vi "test-ltv-differential-drive-controller-Test1.vi"() -> (3 "All tests passed":bool)   [LabVIEW 2019]
uses:
  <vilib>/Rock Robotics/WPI/ThirdParty/JAS_Junk/TrajLib/TRAJ_STATE.ctl
  <vilib>/Rock Robotics/WPI/ThirdParty/JAS_Junk/TrajLib/POSE2D.ctl
  <vilib>/Rock Robotics/WPI/ThirdParty/JAS_Junk/TrajLib/TRANSLATION2D.ctl
  <vilib>/Rock Robotics/WPI/ThirdParty/JAS_Junk/TrajLib/ROTATION2D.ctl
  <vilib>/Rock Robotics/WPI/ThirdParty/JAS_Junk/TrajLib/LINEAR_SYSTEM.ctl
  <vilib>/Analysis/Matrix/Datatypes/RealMatrix.ctl
  <vilib>/Rock Robotics/WPI/ThirdParty/JAS_Junk/TrajLib/LTV_DIFF_DRIVE_CTRL.ctl
  <vilib>/Rock Robotics/WPI/ThirdParty/JAS_Junk/TrajLib/FUNCTION_GENERATOR_MATRIX.ctl
  <vilib>/Rock Robotics/WPI/ThirdParty/JAS_Junk/TrajLib/TRAJECTORY_SPLINE_TYPE_ENUM.ctl
  <vilib>/numeric/Random Number (Range) DBL.vi
  <vilib>/Rock Robotics/WPI/ThirdParty/JAS_Junk/TrajLib/Conv_Inches_Meters.vi
  <vilib>/Rock Robotics/WPI/ThirdParty/JAS_Junk/TrajLib/Rotation2d_CreateAngle.vi
  <vilib>/Rock Robotics/WPI/ThirdParty/JAS_Junk/TrajLib/Translation2d_Create.vi
  <vilib>/Rock Robotics/WPI/ThirdParty/JAS_Junk/TrajLib/MatBuilder_Create.vi
  <vilib>/Rock Robotics/WPI/ThirdParty/JAS_Junk/TrajLib/LinearSystem_New.vi
  <vilib>/Rock Robotics/WPI/ThirdParty/JAS_Junk/TrajLib/MatrixHelper_Zero.vi
  <vilib>/Rock Robotics/WPI/ThirdParty/JAS_Junk/TrajLib/MatBuilder_Fill.vi
  <vilib>/Rock Robotics/WPI/ThirdParty/JAS_Junk/TrajLib/MatrixHelper_CoerceSize.vi
  <vilib>/Analysis/Matrix/Numeric/Add/Add - RM,RM.vi
  <vilib>/Rock Robotics/WPI/ThirdParty/JAS_Junk/TrajLib/Trajectory_Library.lvlib
  <vilib>/Analysis/Matrix/NI_Matrix.lvlib
panel:
  out "Error Graph":dbl[][](graph)
  out "DiffDriveCtrl":T1
  out "Output":T3
  out "Return X":T3
  out "Time":dbl=-1.0
  out "Create Error":bool
  out "Linearsystem":T4
  out "Error":bool
  out "Max\nIterationCount":i32
  out "Any Calc Error":bool
  out "Output Graph":dbl[][](graph)
  out "XY Graph":cluster{dbl[], dbl[]}[](graph)
  out "X":bool
  out "Y":bool
  out "Rot":bool
  out "TotalTime_Sec":dbl
  out "Calc Error":bool
  out "TrajStatePose":T5={"TRANSLATION"={"X"=0.0, "Y"=0.0}, "ROTATION"={"VALUE"=0.0, "COS"=1.0, "SIN"=0.0}} {"ROTATION"."SIN" format="%13.4f"; "ROTATION"."COS" format="%13.4f"; "ROTATION"."VALUE" format="%13.4f"; "TRANSLATION"."Y" format="%14.3f"; "TRANSLATION"."X" format="%14.3f"}
  out "UpdatedPose":T5 {"ROTATION"."SIN" format="%13.4f"; "ROTATION"."COS" format="%13.4f"; "ROTATION"."VALUE" format="%13.4f"; "TRANSLATION"."Y" format="%14.3f"; "TRANSLATION"."X" format="%14.3f"}
  out "OutputTRAJ_STATE":T8={"TimeSeconds"=0.0, "Velocity"=0.0, "Acceleration"=0.0, "POSE"={"TRANSLATION"={"X"=0.0, "Y"=0.0}, "ROTATION"={"VALUE"=0.0, "COS"=1.0, "SIN"=0.0}}, "Curvature"=0.0} {"POSE"."ROTATION"."SIN" format="%13.4f"; "POSE"."ROTATION"."COS" format="%13.4f"; "POSE"."ROTATION"."VALUE" format="%13.4f"; "POSE"."TRANSLATION"."Y" format="%14.3f"; "POSE"."TRANSLATION"."X" format="%14.3f"}
  out "At Reference":bool
  in  "Use Noise":bool
  in  "Use Output Limit":bool=TRUE
  # "< 5, 1 >"
  # "< 2 1 >"
  # "<States,States>"
  # "<States,Inputs>"
  # "<Outputs,States>"
  # "<Outputs,Inputs>"
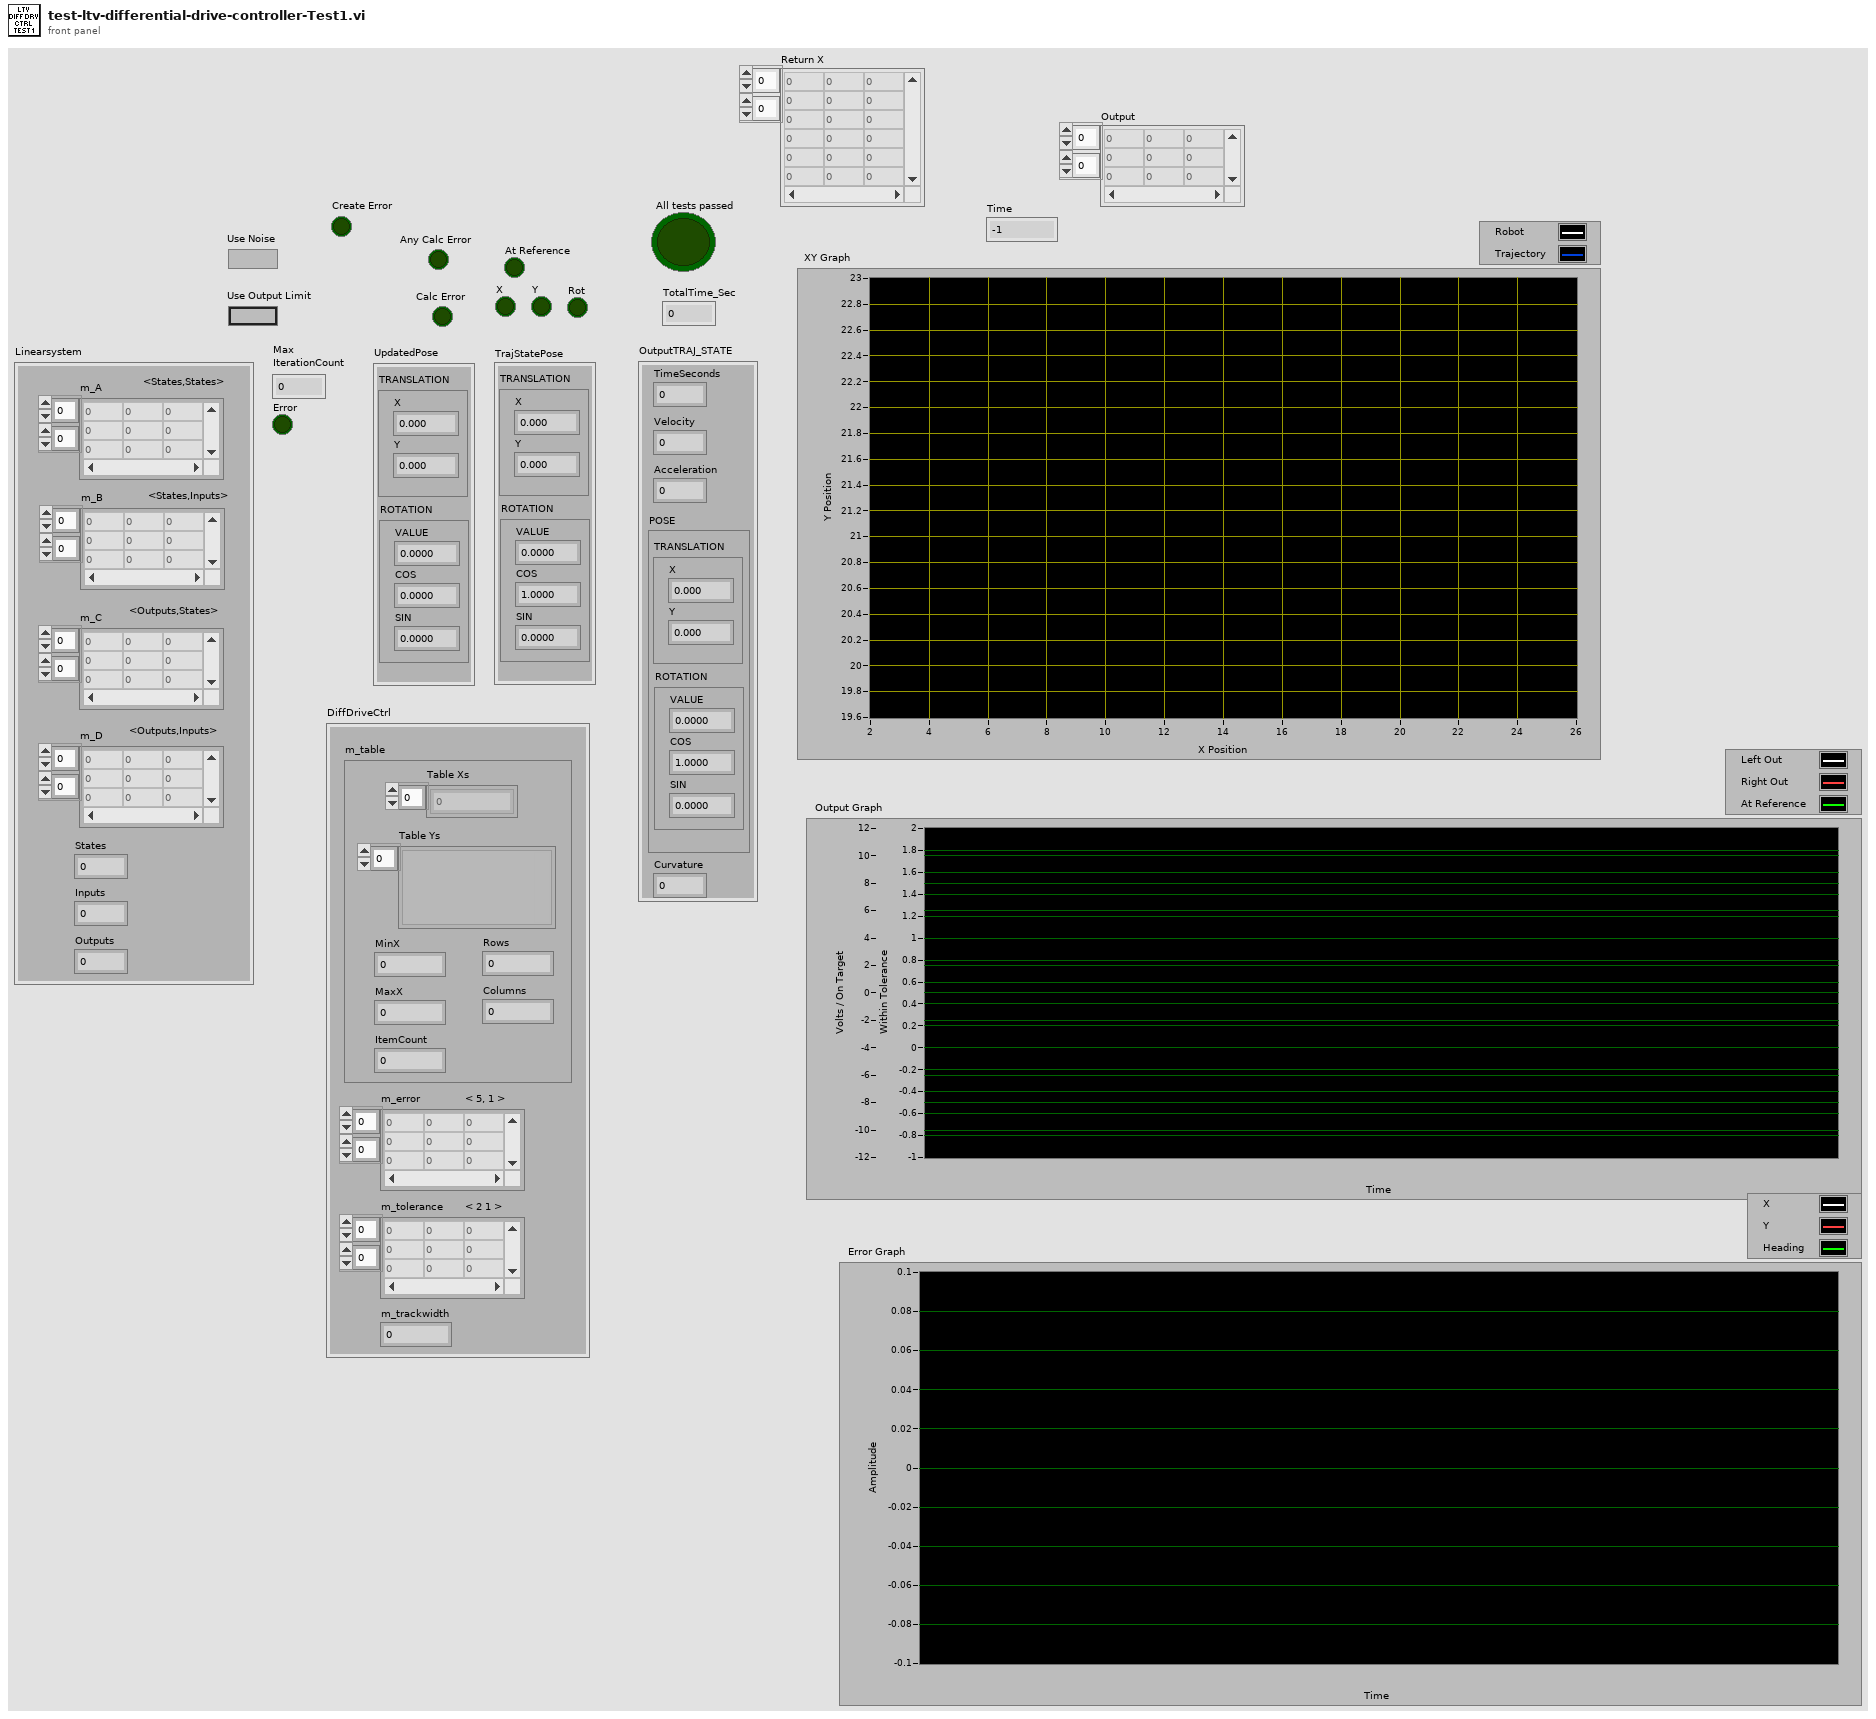
[diagram p1: front panel]
types:
  T1 = typedef "Trajectory_Library.lvlib/LTV_DIFF_DRIVE_CTRL.ctl" = cluster{"m_table":T2, "m_error":T3, "m_tolerance":T3, "m_trackwidth":dbl}
  T2 = typedef "Trajectory_Library.lvlib/FUNCTION_GENERATOR_MATRIX.ctl" = cluster{"Table Xs":dbl[], "Table Ys":variant[], "MinX":dbl, "MaxX":dbl, "ItemCount":i32, "Rows":i32, "Columns":i32}
  T3 = typedef "NI_Matrix.lvlib/RealMatrix.ctl" = dbl[][]
  T4 = typedef "Trajectory_Library.lvlib/LINEAR_SYSTEM.ctl" = cluster{"m_A":T3, "m_B":T3, "m_C":T3, "m_D":T3, "States":i32, "Inputs":i32, "Outputs":i32}
  T5 = typedef "Trajectory_Library.lvlib/POSE2D.ctl" = cluster{"TRANSLATION":T6, "ROTATION":T7}
  T6 = typedef "Trajectory_Library.lvlib/TRANSLATION2D.ctl" = cluster{"X":dbl, "Y":dbl}
  T7 = typedef "Trajectory_Library.lvlib/ROTATION2D.ctl" = cluster{"VALUE":dbl, "COS":dbl, "SIN":dbl}
  T8 = typedef "Trajectory_Library.lvlib/TRAJ_STATE.ctl" = cluster{"TimeSeconds":dbl, "Velocity":dbl, "Acceleration":dbl, "POSE":T5, "Curvature":dbl}
  T9 = typedef "Trajectory_Library.lvlib/TRAJECTORY_SPLINE_TYPE_ENUM.ctl" = enum16{"Cubic", "Cubic With Weights", "Quintic", "Quintic With Weights"}
  T10 = typedef "Trajectory_Library.lvlib/WEIGHTED_WAYPOINT.ctl" = cluster{"TRANSLATION":T6, "ROTATION":T7, "SCALAR":dbl}
  T11 = typedef "Trajectory_Library.lvlib/TRAJ_CONFIG.ctl" = cluster{"MaxVelocity":dbl, "Max Acceleration":dbl, "StartVelocity":dbl, "End Velocity":dbl, "Reversed":bool, "DiffDrKineConstntDefined":bool, "CentAcellConstntDefined":bool, "DiffDrVoltConstntDefined":bool, "DIFF_DRIVE_KINE_CONSTRAINT":T12, "CENTRIPETAL_ACCEL_CONSTRAINT":T14, "SwerveDrKineConstntDefined":bool, "SWERVE_DRIVE_KINE_CONSTRAINT":T15, "DIFF_DRIVE_VOLTAGE_CONSTRAINT":T17, "MECANUM_DRIVE_KINE_CONSTRAINT":T19, "MecanumDrKineConstntDefined":bool}
  T12 = typedef "Trajectory_Library.lvlib/TRAJ_CONSTRAINT_DIIF_DRIVE_KINEMATICS.ctl" = cluster{"Max Speed (M/S)":dbl, "DIFF_DRIVE_KINEMATICS":T13, "Max Accel (M/S2)":dbl}
  T13 = typedef "Trajectory_Library.lvlib/DIFF_DRIVE_KINEMATICS.ctl" = cluster{"TrackWidth_Meters":dbl}
  T14 = typedef "Trajectory_Library.lvlib/TRAJ_CONSTRAINT_CENTRIPETAL_ACCEL.ctl" = cluster{"Max Cent Accel":dbl}
  T15 = typedef "Trajectory_Library.lvlib/TRAJ_CONSTRAINT_SWERVE_DRIVE_KINEMATICS.ctl" = cluster{"Max Speed (M/S)":dbl, "SwerveKinematics":T16}
  T16 = typedef "Trajectory_Library.lvlib/SWERVE_DRIVE_KINEMATICS.ctl" = cluster{"NumModules":i32, "InverseKinematics":T3, "ForwardKinematics":T3, "Modules":T6[], "PrevCoR":T6}
  T17 = typedef "Trajectory_Library.lvlib/TRAJ_CONSTRAINT_DIIF_DRIVE_VOLTAGE.ctl" = cluster{"Max Voltage":dbl, "DIFF_DRIVE_KINEMATICS":T13, "SIMPLE_MOTOR_FF":T18}
  T18 = typedef "Trajectory_Library.lvlib/SIMPLE_MOTOR_FF.ctl" = cluster{"Ks":dbl, "Kv":dbl, "Ka":dbl}
  T19 = typedef "Trajectory_Library.lvlib/TRAJ_CONSTRAINT_MECA_DRIVE_KINEMATICS.ctl" = cluster{"Max Speed (M/S)":dbl, "MECA_DRIVE_KINEMATICS":T20}
  T20 = typedef "Trajectory_Library.lvlib/MECA_DRIVE_KINEMATICS.ctl" = cluster{"FrontLeft":T6, "FrontRight":T6, "RearLeft":T6, "RearRight":T6, "InverseKinematics":T3, "ForwardKinematics":T3, "PrevCoR":T6}
  T21 = typedef "Trajectory_Library.lvlib/TRAJECTORY.ctl" = cluster{"TotalTImeSecs":dbl, "States":T8[]}
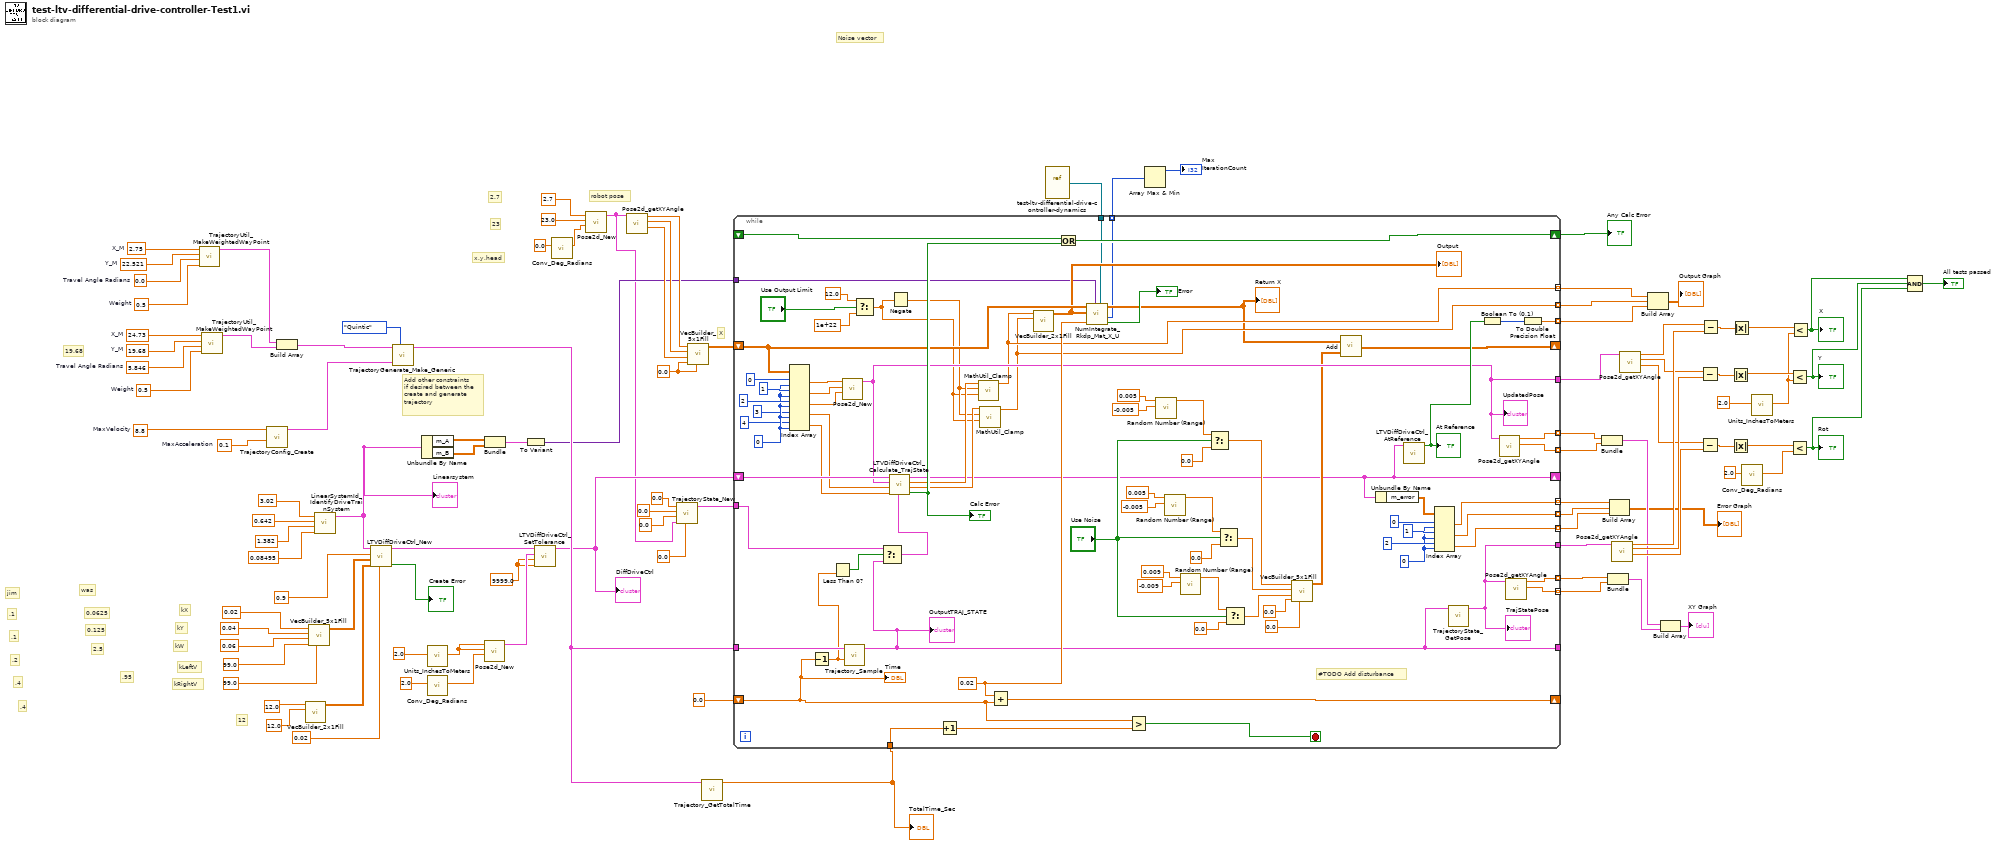
[diagram p0: block diagram]
diagram:
  w15 = 9999.0 ("LeftVelTolerance")
  w30 = 0.0 ("R3")
  w90 = 24.73  # X_M
  w89 = 19.68  # Y_M
  w77 = 5.846  # Travel Angle Radians
  w88 = 0.5  # Weight
  w87 = 2.75  # X_M
  w86 = 22.521  # Y_M
  w78 = 0.0  # Travel Angle Radians
  w85 = 0.5  # Weight
  w84 = 8.8  # MaxVelocity
  w83 = 0.1  # MaxAcceleration
  # "Noise vector"
  # ".4"
  # ".4"
  # ".2"
  # ".1"
  # ".1"
  # "jim"
  # "19.68"
  # ".95"
  # "12"
  # "2.5"
  # "0.125"
  # "0.0625"
  # "was"
  # "X"
  # "23"
  # "2.7"
  # "x,y,head"
  # "robot pose"
  # "Add other constraints\nif desired between the\ncreate and generate\ntrajectory"
  # "kRightV"
  # "kLeftV"
  # "kW"
  # "kY"
  # "kX"
  n1 = call <vilib>:"TrajectoryUtil_MakeWeightedWayPoint.vi"("Weight"=w85, "Travel Angle Radians"=w78, "Y_M"=w86, "X_M"=w87) -> ("WEIGHTED_WAYPOINT"=w79:T10)  [unwired: 7 in]
  n2 = call <vilib>:"TrajectoryUtil_MakeWeightedWayPoint.vi"("Weight"=w88, "Travel Angle Radians"=w77, "Y_M"=w89, "X_M"=w90) -> ("WEIGHTED_WAYPOINT"=w91:T10)  [unwired: 7 in]
  n3 = call <vilib>:"TrajectoryConfig_Create.vi"("MaxAcceleration"=w83, "MaxVelocity"=w84) -> ("TRAJECTORY_CONFIG"=w82:T11)  [unwired: 9 in]
  n4 = Build Array(w79, w91) -> (w80:T10[])
  n5 = call <vilib>:"VecBuilder_2x1Fill.vi"("R1"=12.0, "R0"=12.0) -> ("output matrix"=w70:T3)  [unwired: 9 in]
  n6 = call <vilib>:"VecBuilder_5x1Fill.vi"("R4"=99.0, "R3"=99.0, "R2"=0.06, "R1"=0.04, "R0"=0.02) -> ("output matrix"=w71:T3)  [unwired: 6 in]
  n7 = call <vilib>:"LinearSystemId_IdentifyDriveTrainSystem.vi"("kAAngular"=0.08495, "kVAngular"=1.382, "kALinear"=0.642, "kVLinear"=3.02) -> ("Linearsystem"=w24:T4)  [unwired: 6 in, 1 out]
  "Linearsystem" <- w24
  n8 = call <vilib>:"LTVDiffDriveCtrl_New.vi"("dT"=0.02, "Relms"=w70, "Qelms"=w71, "TrackWidth"=0.9, "Plant"=w24) -> ("Error"=→"Create Error":bool, "DiffDriveCtrl"=w18:T1)  [unwired: 4 in, 1 out]
  n9 = call <vilib>:"TrajectoryGenerate_Make_Generic.vi"("Spline Type"=TRAJECTORY_SPLINE_TYPE_ENUM."Quintic", "traj_config"=w82, "WeightedWayPoints"=w80) -> ("TRAJECTORY"=w67:T21)  [unwired: 7 in, 1 out]
  n10 = Unbundle By Name(w24) -> ("m_A"=w28:T3, "m_B"=w27:T3)
  n11 = call <vilib>:"Units_InchesToMeters.vi"("Inches"=2.0 ("x")) -> ("Meters"=w20:dbl)  [unwired: 10 in]
  n12 = call <vilib>:"Conv_Deg_Radians.vi"("Degress"=2.0) -> ("Radians"=w19:dbl)  [unwired: 10 in]
  n13 = call <vilib>:"Pose2d_New.vi"("Heading"=w19, "Y"=w20, "X"=w20) -> ("out POSe"=w16:T5)  [unwired: 8 in]
  n14 = Bundle("m_A"=w28, "m_B"=w27) -> (w26:cluster{"m_A":T3, "m_B":T3})  [unwired: 1 in]
  n15 = To Variant(anything=w26) -> (Variant=w25:variant)
  n16 = call <vilib>:"LTVDiffDriveCtrl_SetTolerance.vi"("RightVelTolerance"=w15, "LeftVelTolerance"=w15, "PoseTolerance"=w16, "in LTV_DIFF_DRIVE_CONTROLLER"=w18) -> ("out LTV_DIFF_DRIVE_CONTROLLER"=w17:T1)  [unwired: 7 in]
  "DiffDriveCtrl" <- w17
  n17 = call <vilib>:"Conv_Deg_Radians.vi"("Degress"=0.0) -> ("Radians"=w76:dbl)  [unwired: 10 in]
  n18 = call <vilib>:"Pose2d_New.vi"("Heading"=w76, "Y"=23.0, "X"=2.7) -> ("out POSe"=w3:T5)  [unwired: 8 in]
  n19 = call <vilib>:"Pose2d_getXYAngle.vi"("in POSE"=w3) -> ("Angle"=w31:dbl, "Y"=w32:dbl, "X"=w33:dbl)  [unwired: 8 in]
  n20 = call <vilib>:"TrajectoryState_New.vi"("Curvature"=0.0, "POSE"=w3, "Accel"=0.0, "Velocity"=0.0, "Time"=0.0) -> ("TRAJ_STATE"=w1:T8)  [unwired: 6 in]
  n21 = call <vilib>:"VecBuilder_5x1Fill.vi"("R4"=w30, "R3"=w30, "R2"=w31, "R1"=w32, "R0"=w33) -> ("output matrix"=w34:T3)  [unwired: 6 in]
  n22 = call <vilib>:"Trajectory_GetTotalTime.vi"("TRAJECTORY"=w67) -> ("TotalTime_Sec"=w68:dbl)  [unwired: 10 in]
  "TotalTime_Sec" <- w68
  n23 = vi-ref "test-ltv-differential-drive-controller-dynamics.vi"() -> (w29:refnum<vi>)
  n24 = while {
    shift-right: [w183] -> _
    shift-left: 0.0 -> [w109]
    tunnel: w68 -> [w163]
    tunnel: w67 -> [w182]
    shift-right: [w121] -> _
    shift-left: w34 -> [w148]
    shift-right: [w118] -> _
    shift-left: w17 -> [w161]
    tunnel: [w108] -> _
    tunnel: [w177] -> w41
    tunnel: [w181] -> w40 mode=indexing
    tunnel: [w180] -> w39 mode=indexing
    tunnel: [w179] -> w42 mode=indexing
    tunnel: [w178] -> w43 mode=indexing
    tunnel: [w144] -> w35
    tunnel: [w174] -> w38 mode=indexing
    shift-right: [w168] -> w37
    shift-left: _ -> [w169]
    tunnel: w29 -> [w143]
    tunnel: w25 -> [w142]
    tunnel: [w139] -> w14 mode=indexing
    tunnel: [w138] -> w13 mode=indexing
    tunnel: [w119] -> w12 mode=indexing
    tunnel: [w112] -> w10 mode=indexing
    tunnel: [w111] -> w9 mode=indexing
    tunnel: [w110] -> w8 mode=indexing
    tunnel: w1 -> [w107]
    stop <- w184 stop-if-true
    w114 = 0 ("index (col)")
    w154 = 0 ("index (col)")
    w147 = 0.02 ("x")
    # "#TODO Add disturbance"
    n25 = Index Array(array=w148, index (row) #1=0 ("index (row)"), index (col) #1=w154, index (row) #2=1 ("index (row)"), index (col) #2=w154, index (row) #3=2 ("index (row)"), index (col) #3=w154, index (row) #4=3 ("index (row)"), index (col) #4=w154, index (row) #5=4 ("index (row)"), index (col) #5=w154) -> (element #1=w157:dbl, element #2=w156:dbl, element #3=w155:dbl, element #4=w151:dbl, element #5=w150:dbl)
    n26 = Decrement(x=w109) -> (x-1=w106:dbl)
    n27 = Less Than 0?(x=w106) -> (x < 0?=w105:bool)
    n28 = call <vilib>:"Pose2d_New.vi"("Heading"=w155, "Y"=w156, "X"=w157) -> ("out POSe"=w144:T5)  [unwired: 8 in]
    "UpdatedPose" <- w144
    n29 = call <vilib>:"Trajectory_Sample.vi"("Time"=w106, "InputTRAJECTORY"=w182) -> ("OutputTRAJ_STATE"=w108:T8)  [unwired: 9 in]
    "OutputTRAJ_STATE" <- w108
    n30 = Select(t=12.0, s="Use Output Limit", f=1e+22) -> (s? t:f=w133:dbl)
    n31 = Select(t=w107, s=w105, f=w108) -> (s? t:f=w104:T8)
    n32 = call <vilib>:"LTVDiffDriveCtrl_Calculate_TrajState.vi"("DesiredState"=w104, "Right Velocity"=w150, "Left Velocity"=w151, "CurrentPose"=w144, "in LTVDiffDrveCtrl"=w161) -> ("Error"=w149:bool, "Right Voltage"=w140:dbl, "Left Voltage"=w141:dbl, "out LTVDiffDriveCtrl"=w118:T1)  [unwired: 3 in]
    "Calc Error" <- w149
    n33 = Negate(x=w133) -> (-x=w134:dbl)
    n34 = Increment(x=w163) -> (x+1=w162:dbl)
    n35 = call <vilib>:"MathUtil_Clamp.vi"("High Limit"=w133, "Low Limit"=w134, "Value"=w141) -> ("Result"=w139:dbl)  [unwired: 8 in]
    n36 = call <vilib>:"MathUtil_Clamp.vi"("High Limit"=w133, "Low Limit"=w134, "Value"=w140) -> ("Result"=w138:dbl)  [unwired: 8 in]
    n37 = Add(x=w147, y=w109) -> (x+y=w183:dbl)
    n38 = call <vilib>:"VecBuilder_2x1Fill.vi"("R1"=w138, "R0"=w139) -> ("output matrix"=w146:T3)  [unwired: 9 in]
    "Output" <- w146
    n39 = Or(x=w169, y=w149) -> (x .or. y?=w168:bool)
    n40 = call <vilib>:"NumIntegrate_Rkdp_Mat_X_U.vi"("Func_X_U_Extra"=w143, "PassedData"=w142, "dT_Seconds"=w147, "U"=w146, "X"=w148) -> ("Error"=→"Error":bool, "IterationCount"=w119:i32, "Return X"=w122:T3)  [unwired: 4 in]
    "Return X" <- w122
    n41 = Greater?(x=w109, y=w162) -> (0:w184:bool)
    n42 = call-poly <vilib>:"Random Number (Range).vi"("lower bound (0)"=-0.005, "upper bound (100)"=0.005) -> ("number"=w129:dbl)  [unwired: 9 in]
    n43 = call-poly <vilib>:"Random Number (Range).vi"("lower bound (0)"=-0.005, "upper bound (100)"=0.005) -> ("number"=w166:dbl)  [unwired: 9 in]
    n44 = call-poly <vilib>:"Random Number (Range).vi"("lower bound (0)"=-0.009, "upper bound (100)"=0.009) -> ("number"=w164:dbl)  [unwired: 9 in]
    n45 = Select(t=w129, s="Use Noise", f=0.0) -> (s? t:f=w123:dbl)
    n46 = Select(t=w166, s="Use Noise", f=0.0) -> (s? t:f=w124:dbl)
    n47 = Select(t=w164, s="Use Noise", f=0.0) -> (s? t:f=w125:dbl)
    n48 = call <vilib>:"VecBuilder_5x1Fill.vi"("R4"=0.0, "R3"=0.0, "R2"=w125, "R1"=w124, "R0"=w123) -> ("output matrix"=w120:T3)  [unwired: 6 in]
    n49 = call-poly <vilib>:"Add.vi"("Real Matrix B"=w120, "Real Matrix A"=w122) -> ("A + B"=w121:T3)
    n50 = Unbundle By Name(w118) -> ("m_error"=w113:T3)
    n51 = call <vilib>:"LTVDiffDriveCtrl_AtReference.vi"("LTV_DIFF_DRIVE_CTRL"=w118) -> ("At Reference"=w176:bool)  [unwired: 10 in]
    "At Reference" <- w176
    n52 = Index Array(array=w113, index (row) #1=0 ("index (row)"), index (col) #1=w114, index (row) #2=1 ("index (row)"), index (col) #2=w114, index (row) #3=2 ("index (row)"), index (col) #3=w114) -> (element #1=w112:dbl, element #2=w111:dbl, element #3=w110:dbl)
    n53 = call <vilib>:"TrajectoryState_GetPose.vi"("TRAJ_STATE"=w108) -> ("TrajStatePose"=w177:T5)  [unwired: 10 in]
    "TrajStatePose" <- w177
    n54 = Boolean To (0,1)(Boolean=w176) -> (0, 1=w175:i16)
    n55 = call <vilib>:"Pose2d_getXYAngle.vi"("in POSE"=w144) -> ("Y"=w180:dbl, "X"=w181:dbl)  [unwired: 8 in, 1 out]
    n56 = call <vilib>:"Pose2d_getXYAngle.vi"("in POSE"=w177) -> ("Y"=w178:dbl, "X"=w179:dbl)  [unwired: 8 in, 1 out]
    n57 = To Double Precision Float(number=w175) -> (double precision float=w174:dbl)
    "Time" <- w109
  }
  "Any Calc Error" <- w37
  n58 = Array Max & Min(array=w12) -> (max value=→"Max\nIterationCount":i32)  [unwired: 3 out]
  n59 = Bundle(w40, w39) -> (w52:cluster{dbl[], dbl[]})  [unwired: 1 in]
  n60 = Bundle(w42, w43) -> (w51:cluster{dbl[], dbl[]})  [unwired: 1 in]
  n61 = Build Array(w10, w9, w8) -> (→"Error Graph":dbl[][])
  n62 = call <vilib>:"Pose2d_getXYAngle.vi"("in POSE"=w41) -> ("Angle"=w55:dbl, "Y"=w57:dbl, "X"=w63:dbl)  [unwired: 8 in]
  n63 = call <vilib>:"Pose2d_getXYAngle.vi"("in POSE"=w35) -> ("Angle"=w56:dbl, "Y"=w58:dbl, "X"=w64:dbl)  [unwired: 8 in]
  n64 = Build Array(w14, w13, w38) -> (→"Output Graph":dbl[][])
  n65 = Build Array(w52, w51) -> (→"XY Graph":cluster{dbl[], dbl[]}[])
  n66 = Subtract(x=w58, y=w57) -> (x-y=w61:dbl)
  n67 = Subtract(x=w56, y=w55) -> (x-y=w59:dbl)
  n68 = Subtract(x=w64, y=w63) -> (x-y=w65:dbl)
  n69 = Absolute Value(x=w61) -> (abs(x)=w62:dbl)
  n70 = Absolute Value(x=w59) -> (abs(x)=w60:dbl)
  n71 = Absolute Value(x=w65) -> (abs(x)=w66:dbl)
  n72 = call <vilib>:"Conv_Deg_Radians.vi"("Degress"=2.0) -> ("Radians"=w53:dbl)  [unwired: 10 in]
  n73 = call <vilib>:"Units_InchesToMeters.vi"("Inches"=2.0 ("x")) -> ("Meters"=w45:dbl)  [unwired: 10 in]
  n74 = Less?(x=w62, y=w45) -> (x < y?=w47:bool)
  "Y" <- w47
  n75 = Less?(x=w60, y=w53) -> (x < y?=w46:bool)
  "Rot" <- w46
  n76 = Less?(x=w66, y=w45) -> (x < y?=w48:bool)
  "X" <- w48
  n77 = Compound Arithmetic op=AND(w48, w47, w46) -> (→"All tests passed":bool)
